vi "DCPower_VoltageConfiguration.vi"(0 "IVI Refnum in":refnum<k15>, 1 "Voltage Value By Channel":dbl[](array[numeric]), 3 "Active Channels on Instrument":bool[](array[boolean]), 4 "Channel Name Array":string[](array[string]), 5 "error in (no error)":errorcluster) -> (10 "All Channel Numbers Array":string[](array[string]), 12 "Active Channel Numbers Array":string[](array[string]), 13 "Active Channel Voltage Array":dbl[](array[numeric]), 14 "IVI Refnum out":refnum<k15>, 15 "Active Channel Names Array":string[](array[string]), 17 "Total Voltage Indicator Array":dbl[](array[numeric]), 18 "Active Channels Indicator Array":bool[](array[boolean]), 19 "error out":errorcluster)   [LabVIEW 2019]
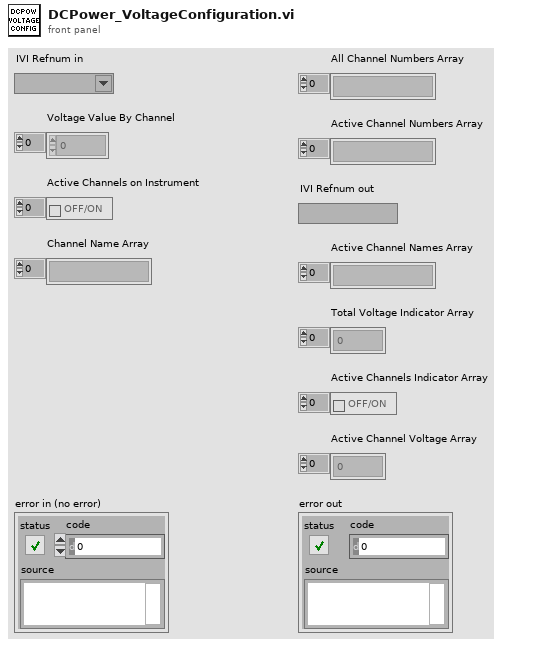
[diagram p1: front panel]
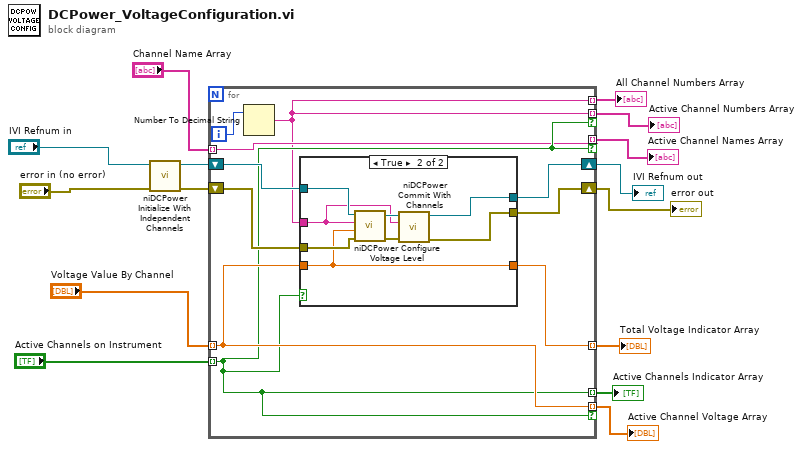
[diagram p0: block diagram]
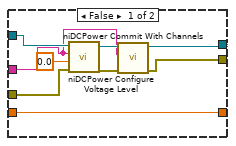
[diagram p2: hidden frame]
diagram:
  n1 = call <instrlib>:"niDCPower Initialize With Independent Channels.vi"("error in (no error)"="error in (no error)", "resource name"="IVI Refnum in") -> ("error out"=w4:errorcluster, "instrument handle out"=w5:refnum<k15>)  [unwired: 8 in]
  n2 = for {
    tunnel: "Active Channels on Instrument" -> [w21] mode=indexing
    shift-right: [w16] -> w1
    shift-left: w4 -> [w23]
    tunnel: "Voltage Value By Channel" -> [w22] mode=indexing
    tunnel: [w21] -> w14 mode=indexing
    tunnel: [w18] -> w11 mode=indexing
    tunnel: [w18] -> w3 mode=indexing if=w21
    tunnel: [w19] -> w12 mode=indexing if=w21
    tunnel: [w22] -> w15 mode=indexing if=w21
    tunnel: [w20] -> w13 mode=indexing
    tunnel: "Channel Name Array" -> [w19] mode=indexing
    shift-right: [w17] -> w2
    shift-left: w5 -> [w24]
    i -> [w25]
    n3 = Number To Decimal String(number=w25) -> (decimal integer string=w18:string)  [unwired: 1 in]
    n4 = case shown="True" w21 {
      tunnel: w24 -> [w32 w41]
      tunnel: w18 -> [w29 w39]
      tunnel: w23 -> [w31 w38]
      tunnel: [w26 w35] -> w16
      tunnel: [w27 w36] -> w17
      tunnel: w22 -> [w28 w37]
      tunnel: [w28 w37] -> w20
      frame False {
        n5 = call <instrlib>:"niDCPower Configure Voltage Level.vi"("error in (no error)"=w31, "voltage level"=0.0, "channel name"=w29, "instrument handle"=w32) -> ("error out"=w34:errorcluster, "instrument handle out"=w30:refnum<k15>)  [unwired: 6 in]
        n6 = call <instrlib>:"niDCPower Commit With Channels.vi"("error in (no error)"=w34, "channel name"=w29, "instrument handle"=w30) -> ("error out"=w26:errorcluster, "instrument handle out"=w27:refnum<k15>)  [unwired: 7 in]
      }
      frame True {
        n7 = call <instrlib>:"niDCPower Configure Voltage Level.vi"("error in (no error)"=w38, "voltage level"=w37, "channel name"=w39, "instrument handle"=w41) -> ("error out"=w42:errorcluster, "instrument handle out"=w40:refnum<k15>)  [unwired: 6 in]
        n8 = call <instrlib>:"niDCPower Commit With Channels.vi"("error in (no error)"=w42, "channel name"=w39, "instrument handle"=w40) -> ("error out"=w35:errorcluster, "instrument handle out"=w36:refnum<k15>)  [unwired: 7 in]
      }
    }
  }
  "Active Channel Voltage Array" <- w15
  "Active Channels Indicator Array" <- w14
  "Total Voltage Indicator Array" <- w13
  "error out" <- w1
  "IVI Refnum out" <- w2
  "Active Channel Names Array" <- w12
  "Active Channel Numbers Array" <- w3
  "All Channel Numbers Array" <- w11
